vi "QWavelength.vi"(8 "error in (no error)":errorcluster, 11 "VISA resource name":refnum<visa-resource-name>) -> (0 "error out":errorcluster, 2 "output":i32, 3 "VISA resource name out":refnum<visa-resource-name>)   [LabVIEW 2009, in "Optical Power meter.lvlib"]
doc: "Returns current wavelength setting"
uses:
  Optical Power meter/Optical Power meter.lvlib
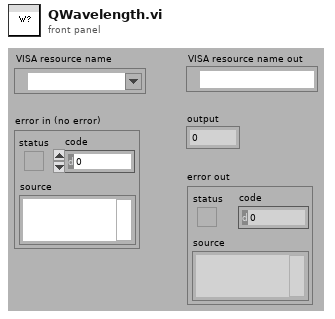
[diagram p1: front panel]
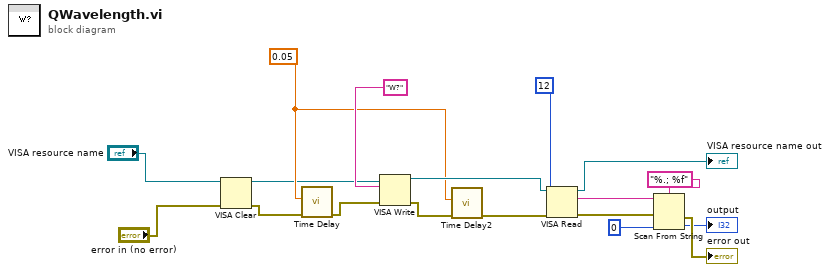
[diagram p0: block diagram]
diagram:
  w8 = 0.05 ("Delay Time (s)")
  n1 = VISA Clear(VISA resource name="VISA resource name", error in (no error)="error in (no error)") -> (VISA resource name out=w6:refnum<visa-resource-name>, error out=w7:errorcluster)
  n2 = call "Time Delay"("error in (no error)"=w7, "Delay Time (s)"=w8) -> ("error out"=w5:errorcluster)  [unwired: 9 in]
  n3 = VISA Write(VISA resource name=w6, write buffer="W?" ("command"), error in (no error)=w5) -> (VISA resource name out=w18:refnum<visa-resource-name>, error out=w4:errorcluster)  [unwired: 1 out]
  n4 = call "Time Delay2"("error in (no error)"=w4, "Delay Time (s)"=w8) -> ("error out"=w3:errorcluster)  [unwired: 9 in]
  n5 = VISA Read(VISA resource name=w18, byte count=u32 12, error in (no error)=w3) -> (VISA resource name out=→"VISA resource name out":refnum<visa-resource-name>, read buffer=w14:string, error out=w12:errorcluster)  [unwired: 1 out]
  n6 = Scan From String(format string="%.; %f", input string=w14, error in=w12, default 1=0 ("default value 1")) -> (error out=→"error out":errorcluster, output 1=→"output":i32)  [unwired: 1 in, 2 out]
